vi "Set_If_Last_Document.vi"(8 "error in (no error)":errorcluster caption="entrée d'erreur (pas d'erreur)", 10 "Last document ?":bool, 11 "Firebase Benches en entrée":refnum<class "Firebase AssembledProducts.lvclass">) -> (0 "error out":errorcluster caption="sortie d'erreur", 3 "Firebase Benches en sortie":refnum<class "Firebase AssembledProducts.lvclass">)   [LabVIEW 2020, in "Library Instrument & Equipement.lvlib" / "Library FireBase.lvlib" / "Firebase AssembledProducts.lvclass"]
uses:
  Firebase AssembledProducts.lvclass
  Firebase AssembledProducts.lvclass/Firebase AssembledProducts.ctl
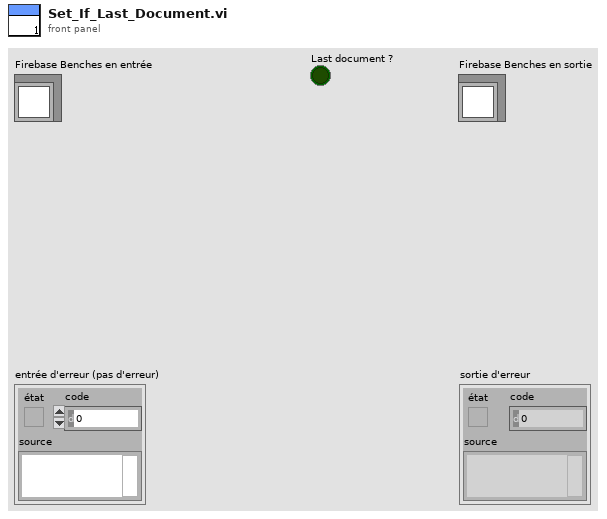
[diagram p1: front panel]
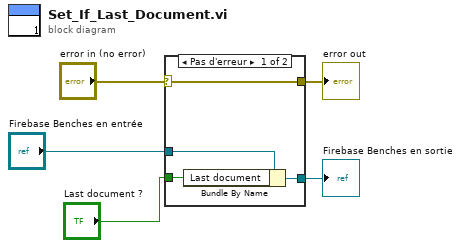
[diagram p0: block diagram]
diagram:
  n1 = case shown="Pas d'erreur" "error in (no error)" {
    selector: "error in (no error)" -> [w9 w11]
    tunnel: [w9 w11] -> w4
    tunnel: [w7 w10] -> w2
    tunnel: "Firebase Benches en entrée" -> [w8 w10]
    tunnel: "Last document ?" -> [w6 _]
    frame No Error {
      n2 = Bundle By Name(cluster=w8, "Last document"=w6) -> (w7:refnum<class "Firebase AssembledProducts.lvclass">)
    }
    frame Error {
    }
  }
  "error out" <- w4
  "Firebase Benches en sortie" <- w2
